vi "RESTful ServiceType To Text.vi"(1 "Service Type":T1) -> (0 "Boolean Text":string)   [LabVIEW 2020]
uses:
  <vilib>/AppBuilder/Engine/RESTful INI Generator/AB_RESTful_ServiceType.ctl
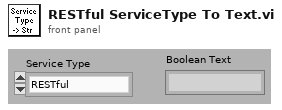
[diagram p1: front panel]
types:
  T1 = typedef "AB_RESTful_ServiceType.ctl" = enum32{"RESTful", "SOAP", "AMQP"}
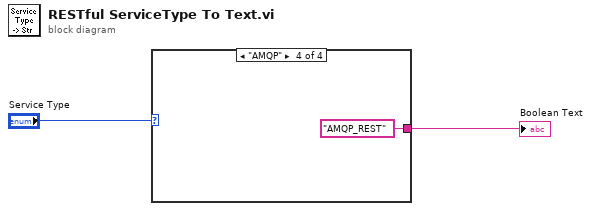
[diagram p0: block diagram]
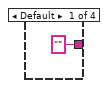
[diagram p2: hidden frame]
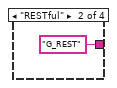
[diagram p3: hidden frame]
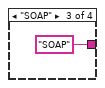
[diagram p4: hidden frame]
diagram:
  n1 = case shown="\"AMQP\"" "Service Type" {
    tunnel: ["" ("Boolean Text") "G_REST" ("Boolean Text") "SOAP" ("Boolean Text") "AMQP_REST" ("Boolean Text")] -> w2
    frame Default {
    }
    frame "RESTful" {
    }
    frame "SOAP" {
    }
    frame "AMQP" {
    }
  }
  "Boolean Text" <- w2
